vi "tester.vi"() -> ()   [LabVIEW 2014]
uses:
  FA_LSSpecialTypes.ctl
  FA_LocalStore.lvlib
panel:
  out "Item XML Output":string[](array[string])
  in  "eTag Value":string="hereisanetag"
  in  "DeleteSpecial Type":T1
  out "eTag Output":string[](array[string])
  out "Error Output":errorcluster[](array[cluster])
  out "Config XML Output":string[](array[string])
  in  "Special Types Array":T1[](array[typedef])
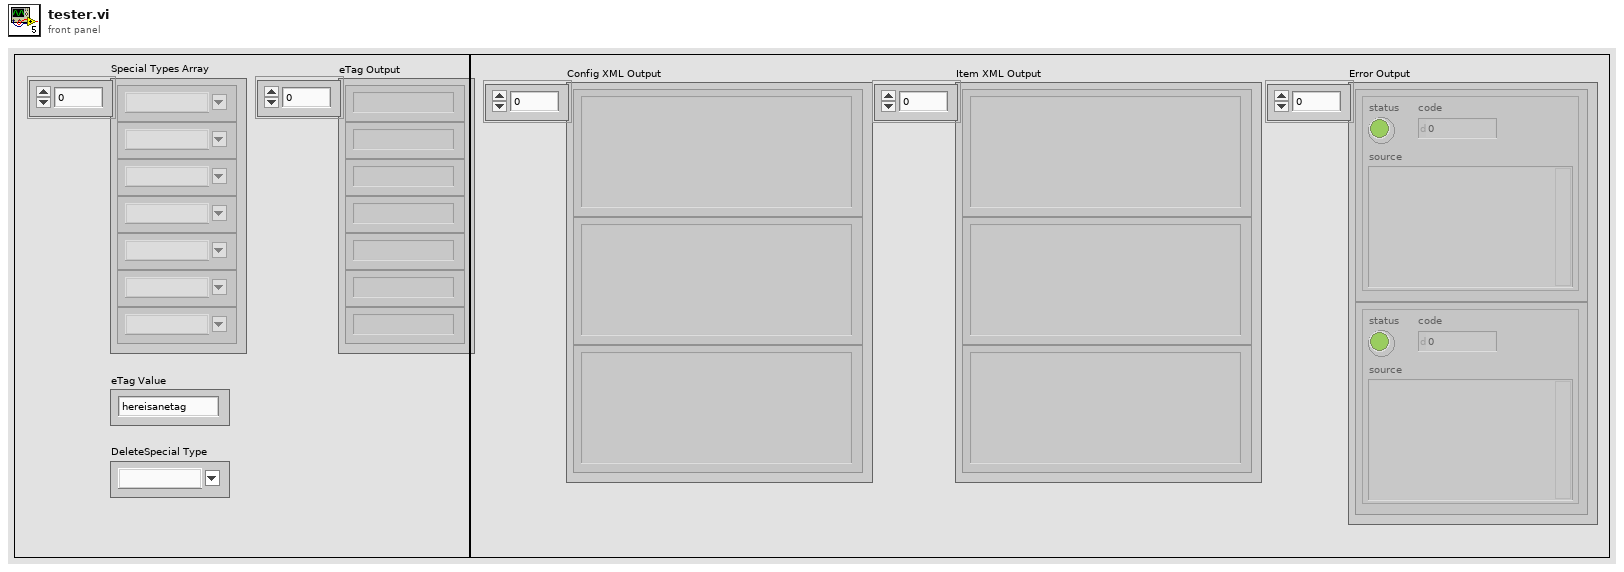
[diagram p1: front panel]
types:
  T1 = typedef "FA_LocalStore.lvlib/FA_LSSpecialTypes.ctl" = string
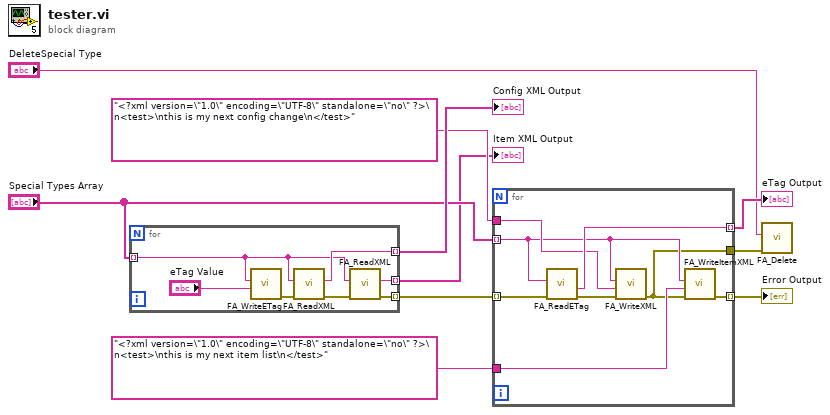
[diagram p0: block diagram]
diagram:
  n1 = for {
    tunnel: [w17] -> w9 mode=indexing
    tunnel: [w13] -> w10 mode=indexing
    tunnel: "Special Types Array" -> [w12] mode=indexing
    tunnel: [w11] -> w1 mode=indexing
    n2 = call "FA_WriteETag.vi"("eTag Value"="eTag Value", "ID"=w12) -> ("Error Out"=w16:errorcluster)  [unwired: 7 in]
    n3 = call "FA_ReadXML.vi"("Error In"=w16, "Special Type"=w12) -> ("Error Out"=w14:errorcluster, "XML String"=w17:string)  [unwired: 6 in]
    n4 = call "FA_ReadXML.vi"("Error In"=w14, "Special Type"=w12) -> ("Error Out"=w13:errorcluster, "XML String"=w11:string)  [unwired: 6 in]
  }
  "Config XML Output" <- w9
  "Item XML Output" <- w1
  n5 = for {
    tunnel: w10 -> [w25] mode=indexing
    tunnel: [w23] -> w8 mode=indexing
    tunnel: "<?xml version=\"1.0\" encoding=\"UTF-8\" standalone=\"no\" ?>\n<test>\nthis is my next config change\n</test>" ("XML String") -> [w22]
    tunnel: "Special Types Array" -> [w20] mode=indexing
    tunnel: "<?xml version=\"1.0\" encoding=\"UTF-8\" standalone=\"no\" ?>\n<test>\nthis is my next item list\n</test>" ("XML String") -> [w21]
    tunnel: [w19] -> w3 mode=indexing
    tunnel: [w18] -> w2
    n6 = call "FA_ReadETag.vi"("Error In"=w25, "ID"=w20) -> ("Error Out"=w24:errorcluster, "ETag"=w23:string)  [unwired: 6 in]
    n7 = call "FA_WriteXML.vi"("Error In"=w24, "XML String"=w22, "Special Type"=w20) -> ("Error Out"=w18:errorcluster)  [unwired: 6 in]
    n8 = call "FA_WriteItemXML.vi"("Error In"=w18, "XML String"=w21, "Special Type"=w20) -> ("Error Out"=w19:errorcluster)  [unwired: 6 in]
  }
  "Error Output" <- w3
  "eTag Output" <- w8
  n9 = call "FA_Delete.vi"("Error In"=w2, "Special Type"="DeleteSpecial Type") -> ()  [unwired: 7 in, 1 out]
